vi "Sort Groups by ID.vi"(8 "error in (no error)":errorcluster, 11 "Transfers Groups in":refnum<class "Transfer Group.lvclass">[](array[class])) -> (0 "error out":errorcluster, 3 "ID-sorted Transfers Groups out":refnum<class "Transfer Group.lvclass">[](array[class]))   [LabVIEW 2017, in "DSF Core.lvlib" / "Transfer Group.lvclass"]
uses:
  Transfer Group.lvclass
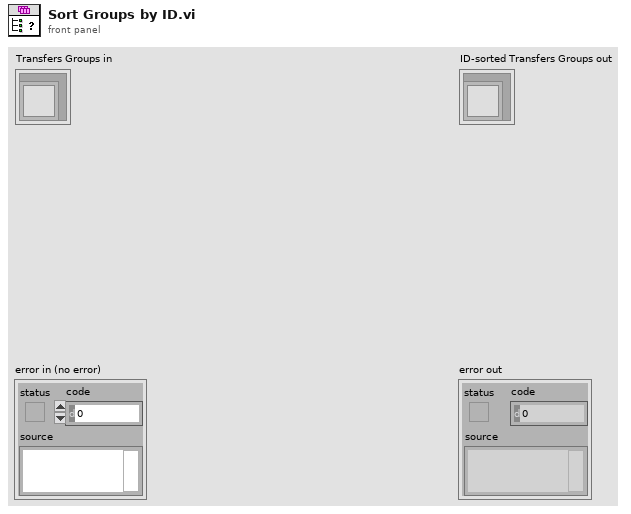
[diagram p1: front panel]
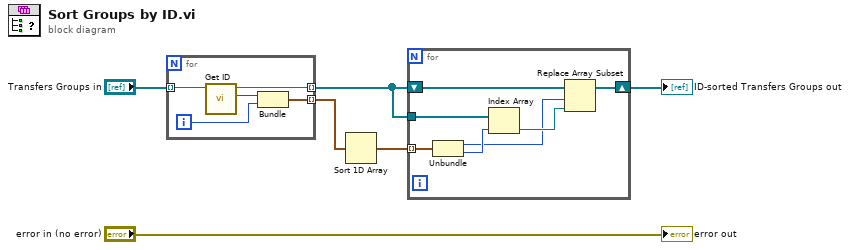
[diagram p0: block diagram]
diagram:
  n1 = for {
    tunnel: "Transfers Groups in" -> [w11] mode=indexing
    tunnel: [w8] -> w3 mode=indexing
    tunnel: [w7] -> w1 mode=indexing
    i -> [w9]
    n2 = call "Get ID.vi"("Transfer Group in"=w11) -> ("id"=w10:i32, "Transfer Group out"=w7:refnum<class "Transfer Group.lvclass">)  [unwired: 9 in]
    n3 = Bundle("id"=w10, w9) -> (w8:cluster{"id":i32, i32})  [unwired: 1 in]
  }
  n4 = Sort 1D Array(array=w3) -> (sorted array=w4:cluster{"id":i32, i32}[])
  n5 = for {
    tunnel: w4 -> [w18] mode=indexing
    shift-right: [w16] -> w2
    shift-left: w1 -> [w17]
    tunnel: w1 -> [w15]
    n6 = Unbundle(w18) -> ("id"=w12:i32, w14:i32)
    n7 = Index Array(array=w15, index=w14) -> (element=w13:refnum<class "Transfer Group.lvclass">)
    n8 = Replace Array Subset(array=w17, new element=w13, index=w12) -> (w16:refnum<class "Transfer Group.lvclass">[])
  }
  "ID-sorted Transfers Groups out" <- w2
  "error out" <- "error in (no error)"
